vi "Initialize.vi"(0 "VISA resource name IN":refnum<visa-resource-name>, 1 "Serial Configuration":T1={"Baud Rate"=9600, "Parity"=2, "Data Bits"=8, "Flow Control"=0} {"Flow Control" items=["None", "XON/XOFF", "RTS/CTS", "XON/XOFF & RTS/CTS"]; "Data Bits" items=["7"=7, "8"=8]; "Parity" items=["None", "Odd", "Even"]; "Baud Rate" items=["1200"=1200, "2400"=2400, "4800"=4800, "9600"=9600, "19200"=19200, "38400"=38400, "57600"=57600, "115200"=115200, "230400"=230400, "460800"=460800, "921600"=921600]}, 2 "User ID (\"\")":string, 5 "ID Query? (True)":bool=TRUE, 7 "Bluetooth Password (\"\")":string, 9 "Serial Auth Type (0: Not Auth)":u16(ring) items=["Not Auth", "RS-232C", "RS-422/485", "Bluetooth"], 11 "error in (no error)":errorcluster, 12 "User Name (\"admin\")":string="admin", 13 "Password (\"\")":string) -> (4 "VISA resource name out":refnum<visa-resource-name>, 15 "error out":errorcluster)   [LabVIEW 2020, in "Yokogawa GX Series.lvlib"]
doc: "Establishes communication with the instrument and optionally performs an instrument identification query. It also places the instrument in a default state needed for other instrument driver operations. Therefore, call this VI before calling other instrument driver VIs for this instrument. Generally, you need to call the <B>Initialize VI</B> only once at the beginning of an application."
uses:
  <instrlib>/Yokogawa GX Series/Yokogawa GX Series.lvlib
panel:
  # "(c) 2013-2018 Yokogawa Electric Corporation.  ALL RIGHTS RESERVED."
  # "Except for TCP/IP or Serial is not supported."
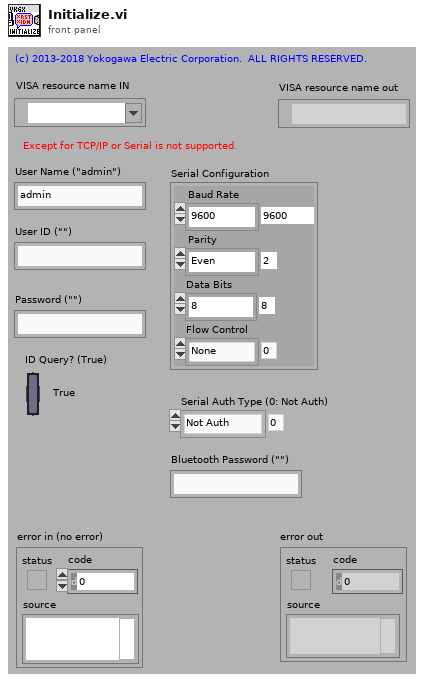
[diagram p1: front panel]
types:
  T1 = cluster{"Baud Rate":u32, "Parity":u16, "Data Bits":u16, "Flow Control":u16}
  T2 = cluster{"Status":bool, "Code":i32, "Source (VI Name)":string}
  T3 = cluster{"User Name":string, "User ID":string, "Password":string, "Serial Auth Type (0: Not Auth)":u16, "SMARTDAC+ Type (0: Unknown)":u16, "Bluetooth Password":string}
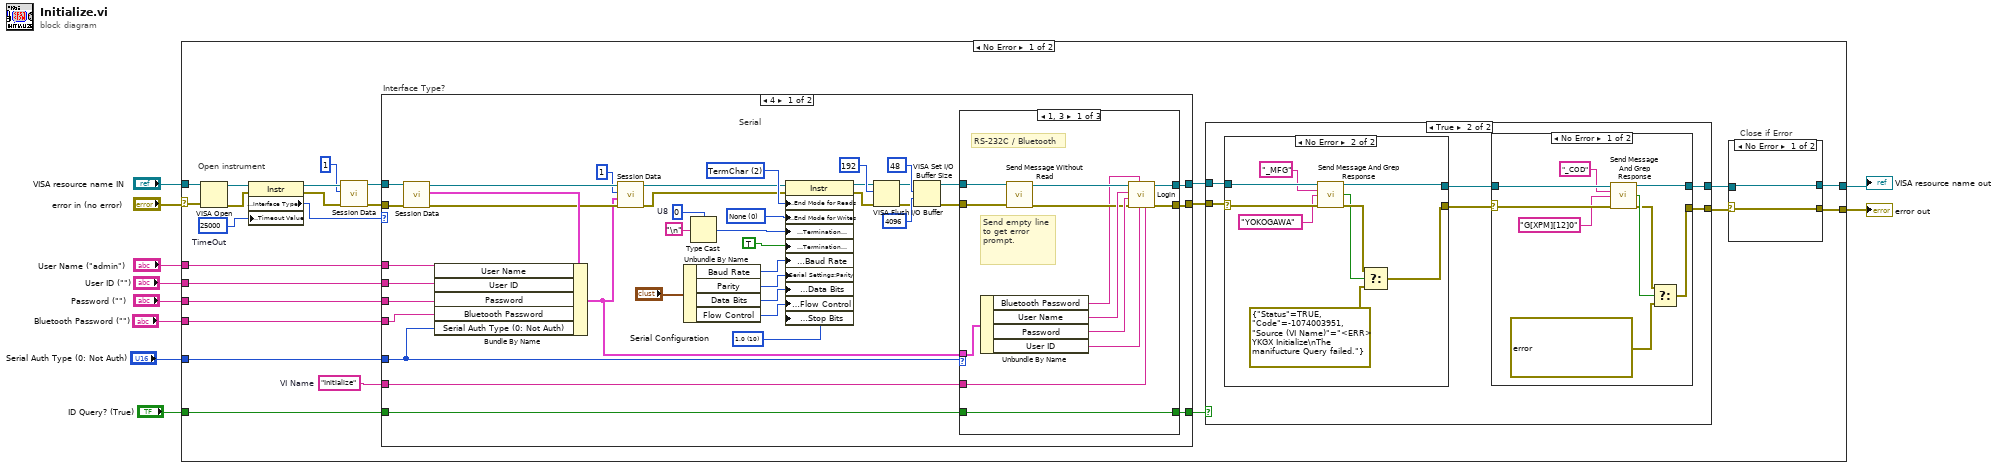
[diagram p0: block diagram]
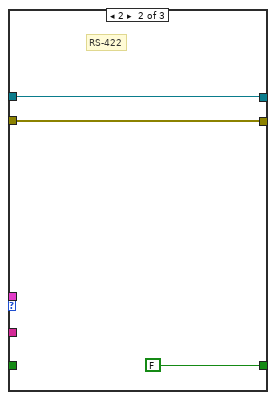
[diagram p5: hidden frame]
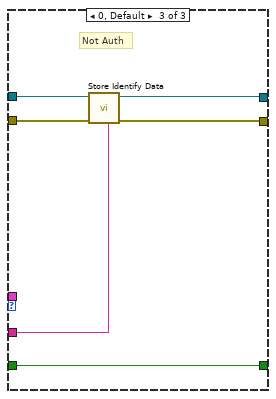
[diagram p6: hidden frame]
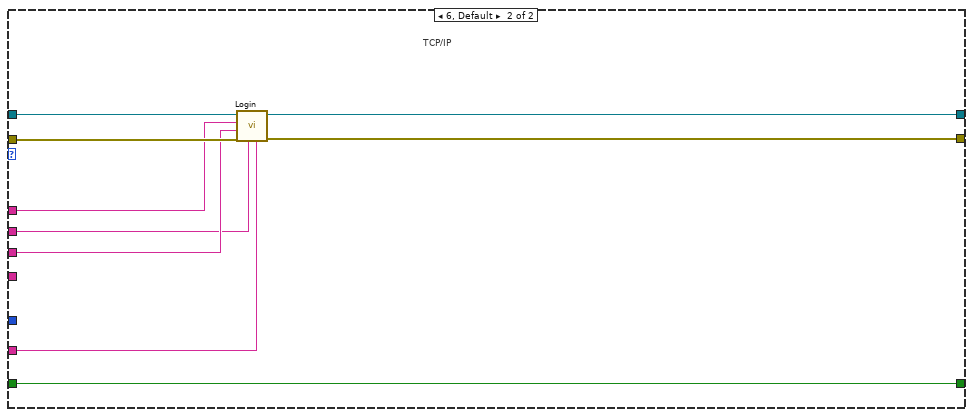
[diagram p7: hidden frame]
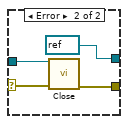
[diagram p8: hidden frame]
diagram:
  n1 = case shown="No Error" "error in (no error)" {
    selector: "error in (no error)" -> [w23 w144]
    tunnel: "User Name (\"admin\")" -> [w34 _]
    tunnel: "Password (\"\")" -> [w33 _]
    tunnel: "VISA resource name IN" -> [w32 w143]
    tunnel: [w27 w143] -> w7
    tunnel: [w24 w144] -> w6
    tunnel: "User ID (\"\")" -> [w20 _]
    tunnel: "Serial Auth Type (0: Not Auth)" -> [w14 _]
    tunnel: "ID Query? (True)" -> [w13 _]
    tunnel: "Bluetooth Password (\"\")" -> [w11 _]
    frame No Error {
      w28 = "Initialize"  # VI Name
      w31 = u32 25000  # TimeOut
      # "Open instrument"
      n2 = VISA Open(error in (no error)=w23, VISA resource name=w32) -> (VISA resource name=w29:refnum<visa-resource-name>, error out=w35:errorcluster)  [unwired: 1 in, 2 out]
      n3 = property class="Instr"(reference=w29, error in=w35, "General Settings:Timeout Value"=w31) -> (reference out=w19:refnum<visa-resource-name>, error out=w18:errorcluster, "Interface Information:Interface Type"=w30:u16)
      n4 = call <instrlib>:"Session Data.vi"("error in (no error)"=w18, "Action (0 : Read Data)"=1, "VISA resource name"=w19) -> ("error out"=w16:errorcluster, "VISA resource name out"=w17:refnum<visa-resource-name>)  [unwired: 6 in, 1 out]
      n5 = case "Interface Type?" shown="4" w30 {
        tunnel: w17 -> [w86 w130]
        tunnel: [w72 w136] -> w26
        tunnel: w16 -> [w85 w133]
        tunnel: [w71 w135] -> w25
        tunnel: w34 -> [w83 w131]
        tunnel: w33 -> [w81 w132]
        tunnel: w28 -> [w70 w134]
        tunnel: w20 -> [w82 w129]
        tunnel: w14 -> [w67 _]
        tunnel: w13 -> [w69 w128]
        tunnel: [w68 w128] -> w12
        tunnel: w11 -> [w66 _]
        frame 4 {
          w98 = u16 10 items=["1.0"=10, "1.5"=15, "2.0"=20] ("Serial Settings:Stop Bits")
          w100 = u16 0 items=["None", "Last Bit", "TermChar", "Break"] ("Serial Settings:End Mode for Writes")
          w101 = u16 2 items=["None", "Last Bit", "TermChar"] ("Serial Settings:End Mode for Reads")
          w104 = u8 0  # U8
          # "Serial"
          n6 = call <instrlib>:"Session Data.vi"("error in (no error)"=w85, "VISA resource name"=w86) -> ("error out"=w79:errorcluster, "User Data Out"=w84:T3, "VISA resource name out"=w80:refnum<visa-resource-name>)  [unwired: 7 in]
          n7 = Bundle By Name(cluster=w84, "User Name"=w83, "User ID"=w82, "Password"=w81, "Bluetooth Password"=w66, "Serial Auth Type (0: Not Auth)"=w67) -> (w73:T3)
          n8 = call <instrlib>:"Session Data.vi"("error in (no error)"=w79, "User Data In"=w73, "Action (0 : Read Data)"=1, "VISA resource name"=w80) -> ("error out"=w76:errorcluster, "VISA resource name out"=w77:refnum<visa-resource-name>)  [unwired: 5 in, 1 out]
          n9 = Unbundle By Name("Serial Configuration") -> ("Baud Rate"=w102:u32, "Parity"=w99:u16, "Data Bits"=w96:u16, "Flow Control"=w88:u16)
          n10 = Type Cast(type=w104, x="\n") -> (*(type *) &x=w87:u8)
          n11 = property class="Instr"(reference=w77, error in=w76, "Serial Settings:End Mode for Reads"=w101, "Serial Settings:End Mode for Writes"=w100, "Message Based Settings:Termination Character"=w87, "Message Based Settings:Termination Character Enable"=TRUE, "Serial Settings:Baud Rate"=w102, "Serial Settings:Parity"=w99, "Serial Settings:Data Bits"=w96, "Serial Settings:Flow Control"=w88, "Serial Settings:Stop Bits"=w98) -> (reference out=w90:refnum<visa-resource-name>, error out=w89:errorcluster)
          n12 = VISA Flush I/O Buffer(VISA resource name=w90, mask (16)=u16 192, error in (no error)=w89) -> (VISA resource name out=w91:refnum<visa-resource-name>, error out=w92:errorcluster)
          n13 = VISA Set I/O Buffer Size(VISA resource name=w91, mask (16)=u16 48, size (4096)=u32 4096 ("size (0)"), error in (no error)=w92) -> (VISA resource name out=w75:refnum<visa-resource-name>, error out=w74:errorcluster)
          n14 = case shown="1, 3" w67 {
            tunnel: w75 -> [w110 w121 w126]
            tunnel: w74 -> [w109 w120 w125]
            tunnel: w73 -> [w118 _ _]
            tunnel: [w117 w121 w124] -> w72
            tunnel: [w116 w120 w123] -> w71
            tunnel: w70 -> [w115 _ w122]
            tunnel: w69 -> [w111 _ w127]
            tunnel: [w111 FALSE w127] -> w68
            frame 1, 3 {
              # "Send empty line to get error prompt."
              # "RS-232C / Bluetooth"
              n15 = Unbundle By Name(w118) -> ("Bluetooth Password"=w106:string, "User Name"=w114:string, "Password"=w113:string, "User ID"=w112:string)
              n16 = call <instrlib>:"Send Message Without Read.vi"("error in (no error)"=w109, "VISA resource name"=w110) -> ("error out"=w107:errorcluster, "VISA resource name out"=w108:refnum<visa-resource-name>)  [unwired: 8 in]
              n17 = call <instrlib>:"Login.vi"("Source (\"\")"=w115, "User ID (\"\")"=w112, "Bluetooth Password (\"\")"=w106, "error in (no error)"=w107, "Password (\"\")"=w113, "User Name (\"admin\")"=w114, "VISA resource name"=w108) -> ("error out"=w116:errorcluster, "VISA resource name out"=w117:refnum<visa-resource-name>)  [unwired: 3 in]
            }
            frame 2 {
              # "RS-422"
            }
            frame 0, Default {
              # "Not Auth"
              n18 = call <instrlib>:"Store Identify Data.vi"("Source (\"\")"=w122, "error in (no error)"=w125, "VISA resource name"=w126) -> ("error out"=w123:errorcluster, "VISA resource name out"=w124:refnum<visa-resource-name>)  [unwired: 7 in]
            }
          }
        }
        frame 6, Default {
          # "TCP/IP"
          n19 = call <instrlib>:"Login.vi"("Source (\"\")"=w134, "User ID (\"\")"=w129, "error in (no error)"=w133, "Password (\"\")"=w132, "User Name (\"admin\")"=w131, "VISA resource name"=w130) -> ("error out"=w135:errorcluster, "VISA resource name out"=w136:refnum<visa-resource-name>)  [unwired: 1 in, 3 out]
        }
      }
      n20 = case shown="True" w12 {
        tunnel: w26 -> [w37 w41]
        tunnel: w25 -> [w36 w40]
        tunnel: [w37 w39] -> w22
        tunnel: [w36 w38] -> w21
        frame False {
        }
        frame True {
          n21 = case shown="No Error" w40 {
            selector: w40 -> [w55 w63]
            tunnel: w41 -> [w56 w60]
            tunnel: [w56 w61] -> w43
            tunnel: [w55 w62] -> w42
            frame Error {
            }
            frame No Error {
              n22 = call <instrlib>:"Send Message And Grep Response.vi"("VISA resource name"=w60, "Command (\"\")"="_MFG", "Strings (\"\")"="YOKOGAWA", "error in (no error)"=w63) -> ("VISA resource name out"=w61:refnum<visa-resource-name>, "Result"=w59:bool, "error out"=w65:errorcluster)  [unwired: 8 in, 1 out]
              n23 = Select(t=w65, s=w59, f=T2 {"Status"=TRUE, "Code"=-1074003951, "Source (VI Name)"="<ERR> YKGX Initialize\nThe manifucture Query failed."}) -> (s? t:f=w62:T2)
            }
          }
          n24 = case shown="No Error" w42 {
            selector: w42 -> [w48 w54]
            tunnel: w43 -> [w49 w53]
            tunnel: [w47 w54] -> w38
            tunnel: [w46 w53] -> w39
            frame No Error {
              n25 = call <instrlib>:"Send Message And Grep Response.vi"("VISA resource name"=w49, "Command (\"\")"="_COD" ("ID query"), "Strings (\"\")"="G[XPM][12]0", "error in (no error)"=w48) -> ("VISA resource name out"=w46:refnum<visa-resource-name>, "Result"=w52:bool, "error out"=w50:errorcluster)  [unwired: 8 in, 1 out]
              n26 = Select(t=w50, s=w52, f=T2 {"Status"=TRUE, "Code"=-1074003951, "Source (VI Name)"="<ERR> YKGX Initialize\nThe ID Query failed.  This may mean that you selected the wrong instrument or your instrument did not respond.  You may also be using a model that is not officially supported by this driver.  If you are sure that you have selected the correct instrument and it is responding, try disabling the ID Query."}) -> (s? t:f=w47:T2)
            }
            frame Error {
            }
          }
        }
      }
      n27 = case "Close if Error" shown="No Error" w21 {
        selector: w21 -> [w138 w141]
        tunnel: w22 -> [w137 w139]
        tunnel: [w137 refnum<visa-resource-name> refnum ("VISA resource name out")] -> w27
        tunnel: [w138 w142] -> w24
        frame No Error {
        }
        frame Error {
          n28 = call <instrlib>:"Close.vi"("error in (no error)"=w141, "VISA resource name"=w139) -> ("error out"=w142:errorcluster)  [unwired: 9 out]
        }
      }
    }
    frame Error {
    }
  }
  "VISA resource name out" <- w7
  "error out" <- w6
